vi "fetch_internet_version.vi"(8 "error in (no error)":errorcluster, 11 "HelioUpdateMH100803 in":refnum<class "HelioUpdateMH100803.lvclass">) -> (0 "error out":errorcluster, 3 "HelioUpdateMH100803 out":refnum<class "HelioUpdateMH100803.lvclass">, 4 "internet version out":string)   [LabVIEW 2010, in "HelioUpdateMH100803.lvclass"]
uses:
  HelioUpdateMH100803.lvclass
  HelioUpdateMH100803.lvclass/HelioUpdateMH100803.ctl
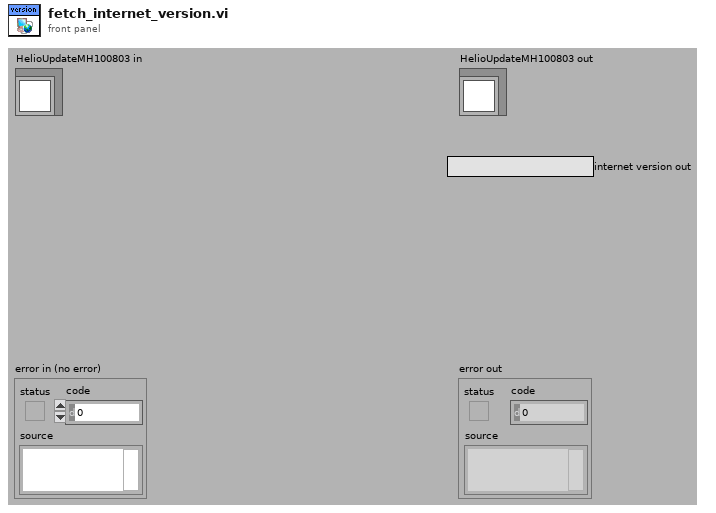
[diagram p1: front panel]
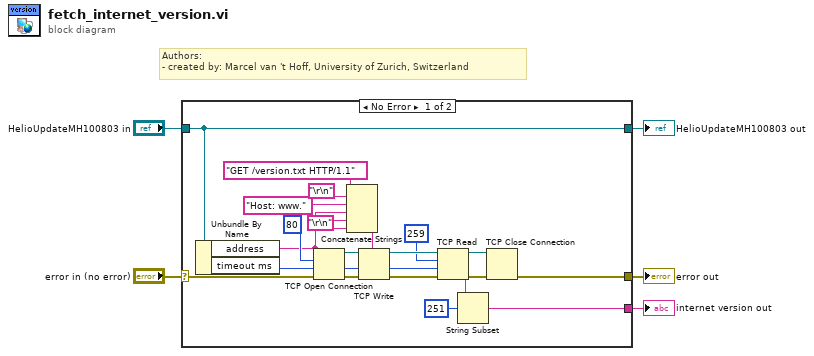
[diagram p0: block diagram]
diagram:
  # "Authors: \n- created by: Marcel van 't Hoff, University of Zurich, Switzerland"
  n1 = case shown="No Error" "error in (no error)" {
    selector: "error in (no error)" -> [w13 w27]
    tunnel: [w10 w27] -> w4
    tunnel: "HelioUpdateMH100803 in" -> [w7 w28]
    tunnel: [w7 w28] -> w3
    tunnel: [w6 _] -> w5
    frame No Error {
      w17 = "\r\n"
      n2 = Unbundle By Name(w7) -> ("address"=w11:string, "timeout ms"=w8:i32)
      n3 = TCP Open Connection(address=w11, remote port or service name=u16 80 ("remote port"), timeout ms (60000)=w8, error in (no error)=w13) -> (connection ID=w12:refnum<k5>, error out=w22:errorcluster)  [unwired: 1 in]
      n4 = Concatenate Strings("GET /version.txt HTTP/1.1" ("data in"), "\r\n", "Host: www." ("string"), w11, w17, w17) -> (w16:string)
      n5 = TCP Write(connection ID=w12, data in=w16, error in (no error)=w22, 9:w8) -> (connection ID out=w26:refnum<k5>, error out=w23:errorcluster)  [unwired: 1 out]
      n6 = TCP Read(connection ID=w26, bytes to read=259, error in (no error)=w23, 9:w8) -> (connection ID out=w24:refnum<k5>, data out=w15:string, error out=w25:errorcluster)  [unwired: 1 out]
      n7 = String Subset(string=w15, offset (0)=251) -> (substring=w6:string)  [unwired: 1 in]
      n8 = TCP Close Connection(connection ID=w24, error in (no error)=w25) -> (error out=w10:errorcluster)  [unwired: 2 out]
    }
    frame Error {
    }
  }
  "error out" <- w4
  "HelioUpdateMH100803 out" <- w3
  "internet version out" <- w5
